vi "Command Injection.vi"() -> ()   [LabVIEW 2023]
doc: "Provides an example implementation of the Hardware Abstraction Framework to allow any attached instrument to be queried for its identity. The instrument must implement the SCPI standard.\n\nThe example application is clearly overly complex for the simple purpose of obtaining identity. However, it has been written to show how complex applications can be derived using the provided Event-Process-Result Handling mechanism. In fact, the base application can be reused by replacing the \"App ActionX Process\" VIs and \"Result Handling VIs\" as needed.\n\nNote that this example is just one way of interacting with the Framework. Ultimately, you just need to set up a Test Processor with what is needed and tell it to \"Process Directors\"."
uses:
  ReadCommand/ReadCommand.lvclass
  All Internal Message Ids.ctl
  ResourceEnumerator/ResourceEnumerator.lvclass
  InteractionProcessor/InteractionProcessor.lvclass
  CommandDirector/CommandDirector.lvclass
  <extravilib>/ChannelInstances/Tag-bool/Read With Abort.vi
  <extravilib>/ChannelInstances/Tag-bool/Write With Abort.vi
  <extravilib>/ChannelInstances/Tag-bool/Instantiate.vi
  <extravilib>/ChannelInstances/Tag-bool/EndpointRead.vi
  <extravilib>/ChannelInstances/Tag-bool/Endpoint.vi
  HAF.lvlib
  <extravilib>/ChannelInstances/Tag-bool.lvlib
panel:
  out "DC Read":u32
  out "DC Write":i32
  out "Read Duty Cycle":i32(slide) min=0 max=4095 step=1 scale=0.0..4095.0
  in  "Set Duty Cycle":i32(slide)=1007 max=4095 step=1 scale=0.0..4095.0
  in  "Pin":u8 max=7 step=1
  out "error out":errorcluster
  out "IDs":string[](array[string])
  out "Running":bool
  in  "Action10":bool
  in  "Action9":bool
  in  "Action8":bool
  in  "Action7":bool
  in  "Action6":bool
  in  "Action5":bool
  in  "Action4":bool
  in  "Action3":bool
  in  "Action2":bool
  in  "Instruments 2":string(combo)
  in  "Resume":bool
  in  "Pause":bool
  in  "Stop":bool
  in  "Start":bool caption="Action1"
  out "Instrument Id":string
  in  "Refresh":bool
  in  "Instruments":string(combo)
  # "Defined Behaviour Buttons"
  # "Command Injection - Pi Pico"
  # "Re-usable Controls\n\nThese are hidden at runtime.  Unhide if used."
  # "Provides an example implementation of the Hardware Abstraction Framework to show how Commands can be injected into an interaction whilst it is already running.  It uses a Raspberry Pi Pico with firmware developed by Jan Cumps and Shabaz available at \nhttps://github.com/jancumps/pico_scpi_usbtmc_labtool/releases/tag/v0.2.1\n\nOnce running, ensure the Pi Pico is selected in the Instruments drop down list then click Start.  Select a pin and move the gauge labelled \"Set Duty Cycle\" to inject commands to write the new value to the Pi and then read the pin. \n\nThe application starts the interaction running with one CommandDirector to get the ID from the Pico.  Normally this would then end the interaction (it's a run-once Director) but the InteractionProcessor is set to Handle Injections which prevents it terminating until Stop is pressed.  Each time the Set Duty Cycle gauge is moved it generates a UI event in the Event Loop which messages the Main Processing Loop to inject the commands.  \n\nThe VI is terminated by clicking on Stop."
  # "Defined Behaviour Buttons\n\nDrag the control from here to where needed.  You can relabel them but their behaviour is fixed in the application.\nYou may change this behaviour as well of course.\nStop and Refresh have been used."
  # "Instruments"
  # "Action Buttons"
  # "Instruments\n\nThese hold a list of Instruments attached to the PC and are populated by the \"Refresh\" Process case.  The Refresh button re-populates them."
  # "Action  Buttons\n\nDrag the control from here to where you need them on your panel.  Re-label and add button text as desired.\n\nPut processing code in the Process Case under their caption value.\n\nAction1 has been used and named \"Get Id\""
  # "="
  # "Other"
  # "Other\n\nOther potentially useful controls or indicators. \nIDs is the collection of UUIDs generated for Commands during execution.\nThe LED Running is used in this example."
  # "="
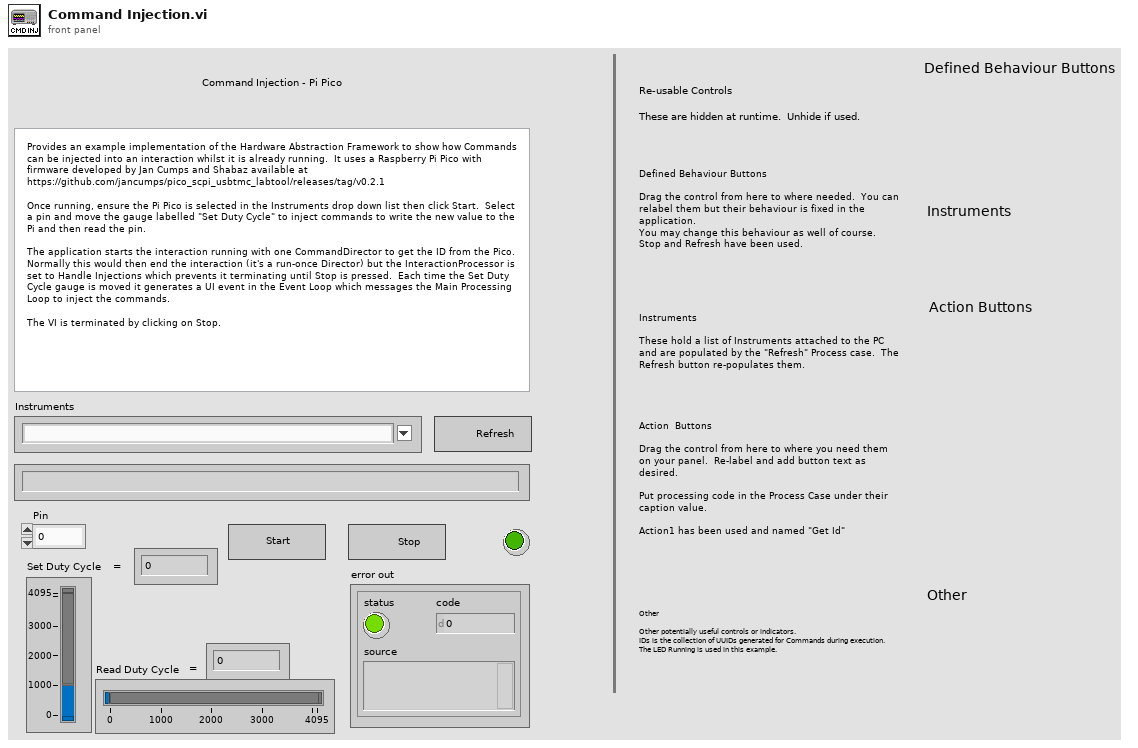
[diagram p1: front panel]
types:
  T1 = typedef "HAF.lvlib/All Message Queues.ctl" = cluster{"Internal":refnum<queue>, "Notifications":refnum<queue>}
  T2 = typedef "HAF.lvlib/All Events.ctl" = cluster{"Stop":T3, "Pause":T4, "Resume":T5, "Done":T6, "Injection":T7}
  T3 = typedef "HAF.lvlib/Stop Event.ctl" = refnum<user-event>
  T4 = typedef "HAF.lvlib/Pause Event.ctl" = refnum<user-event>
  T5 = typedef "HAF.lvlib/Resume Event.ctl" = refnum<user-event>
  T6 = typedef "HAF.lvlib/Done Event.ctl" = refnum<user-event>
  T7 = typedef "HAF.lvlib/Injection Event.ctl" = refnum<user-event>
  T8 = typedef "HAF.lvlib/All Internal Message Ids.ctl" = cluster{"Initialise":string, "Process":string, "Continue":string, "Done":string, "Pause":string, "Resume":string, "Stop":string, "Exit":string, "Inject":string}
  T9 = typedef "Tag-bool.lvlib/))Channel.ctl" = refnum<queue>
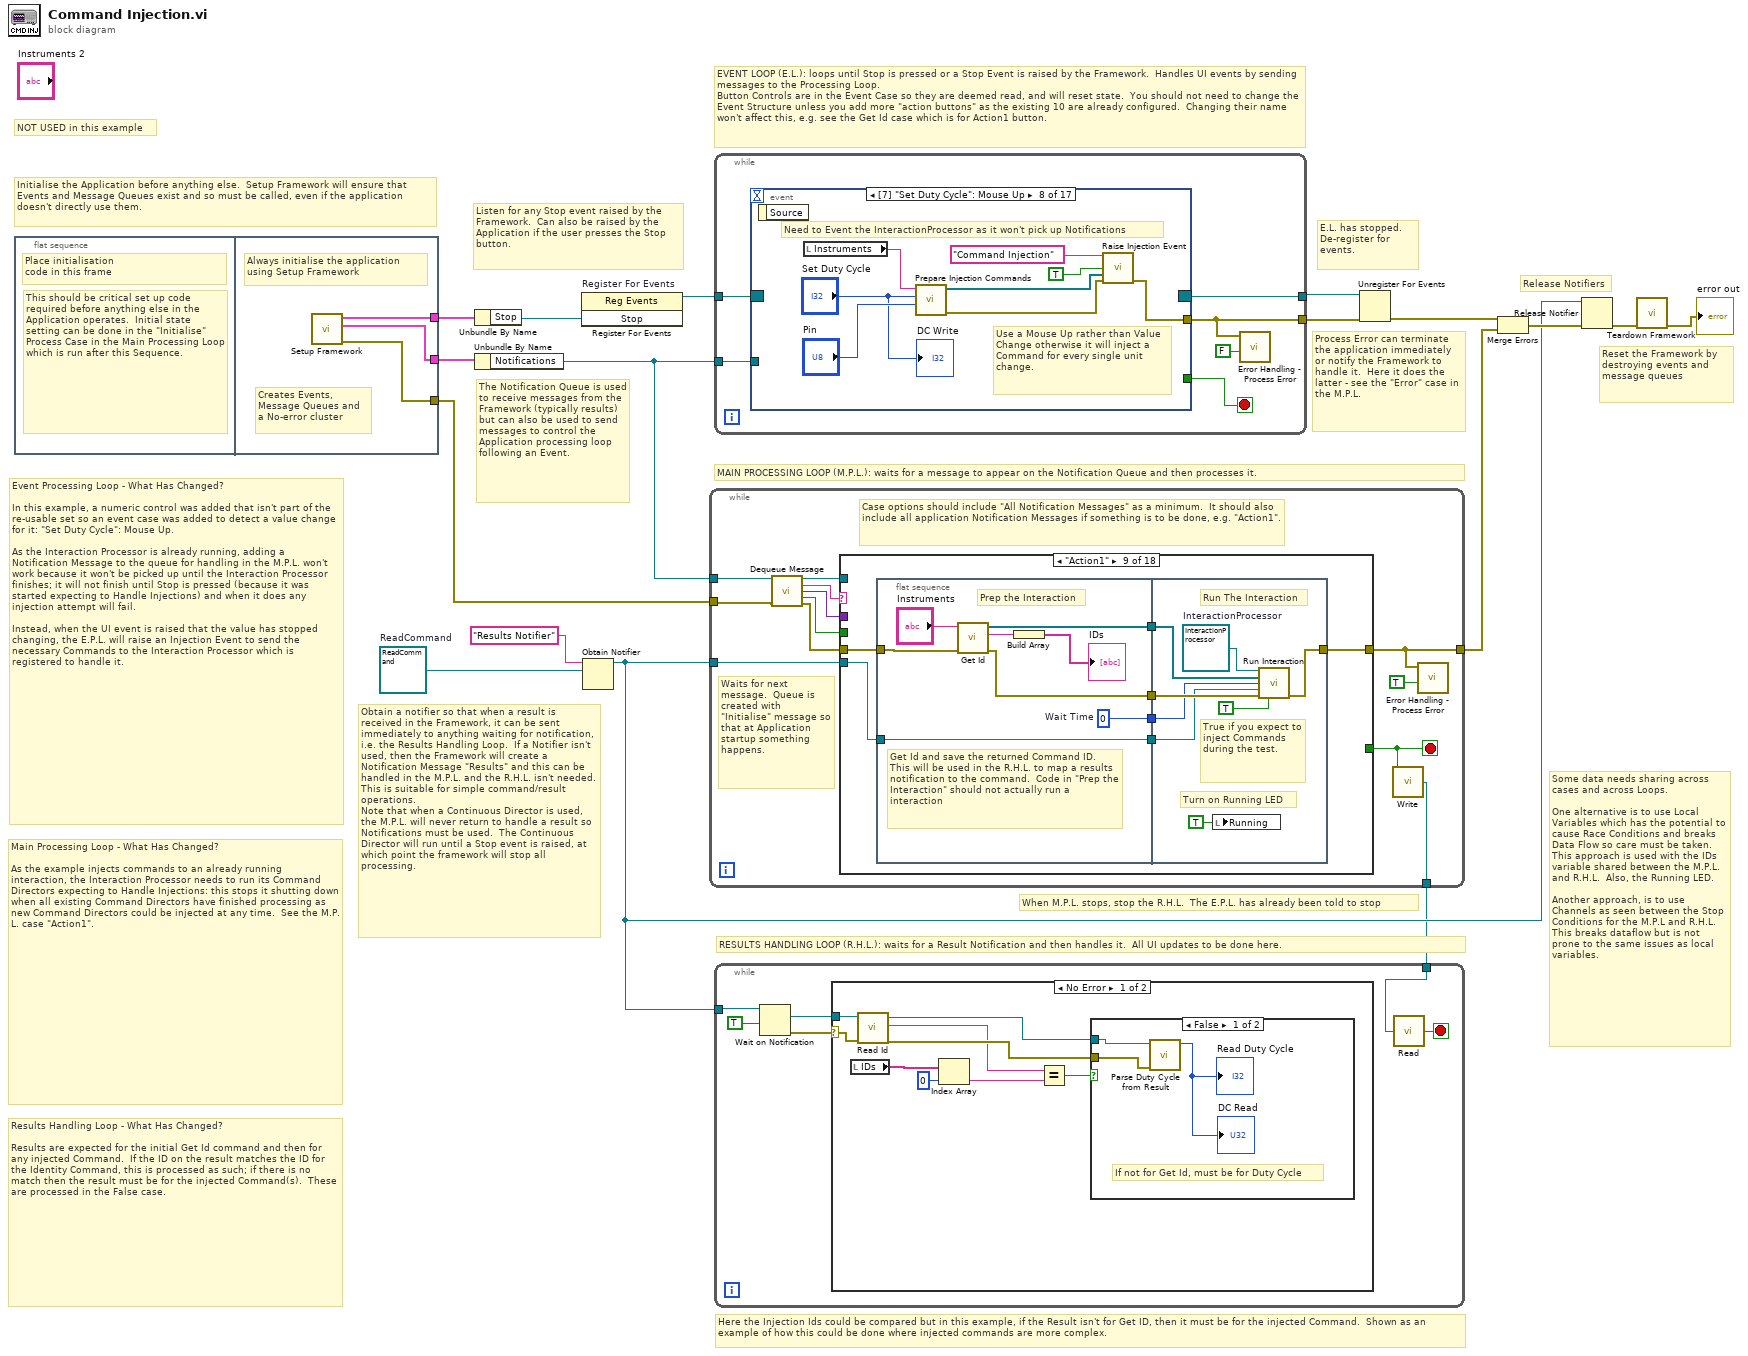
[diagram p0: block diagram]
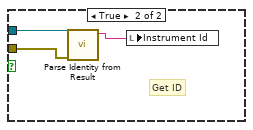
[diagram p2: hidden frame]
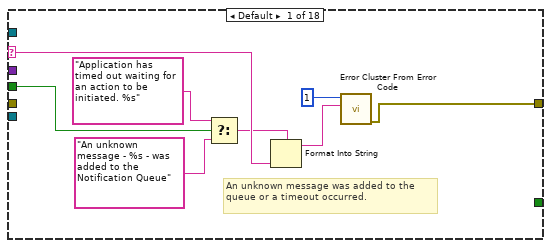
[diagram p4: hidden frame]
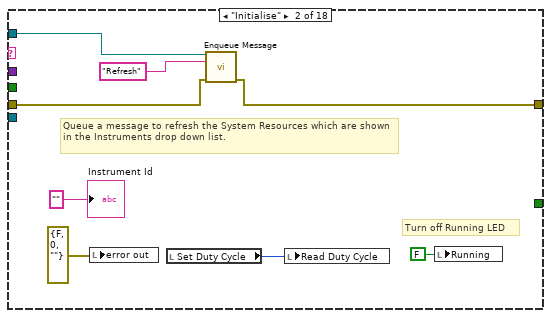
[diagram p5: hidden frame]
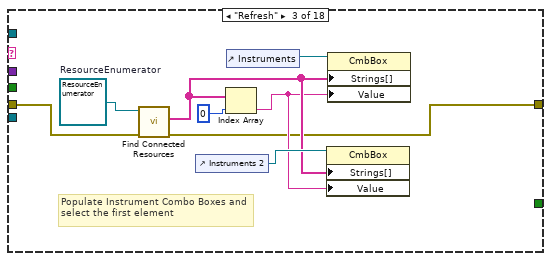
[diagram p6: hidden frame]
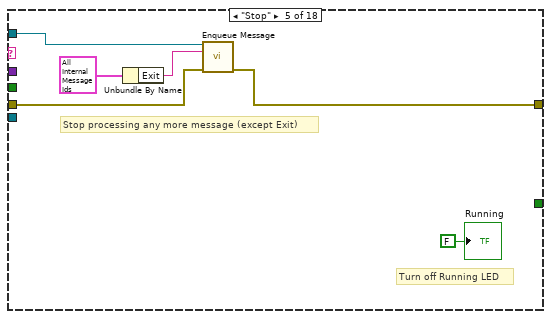
[diagram p8: hidden frame]
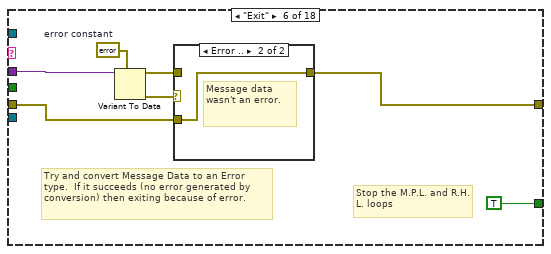
[diagram p9: hidden frame]
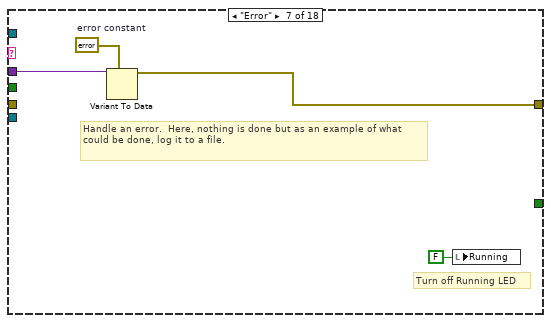
[diagram p11: hidden frame]
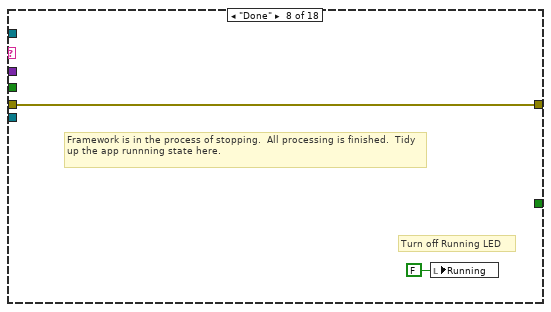
[diagram p12: hidden frame]
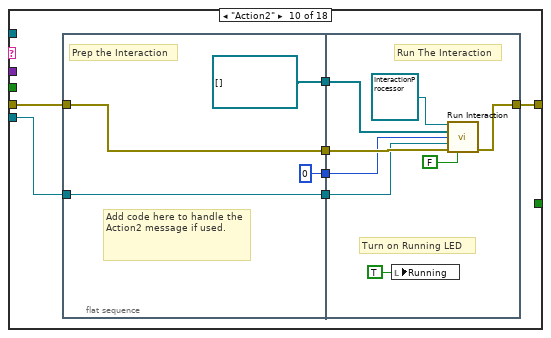
[diagram p13: hidden frame]
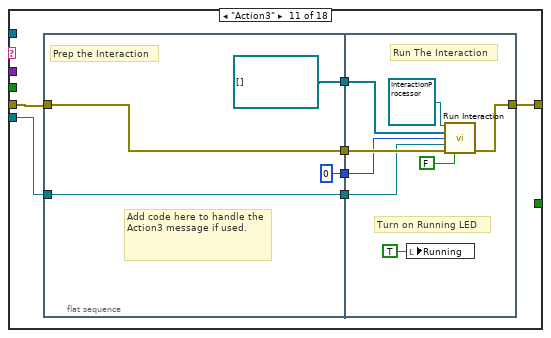
[diagram p14: hidden frame]
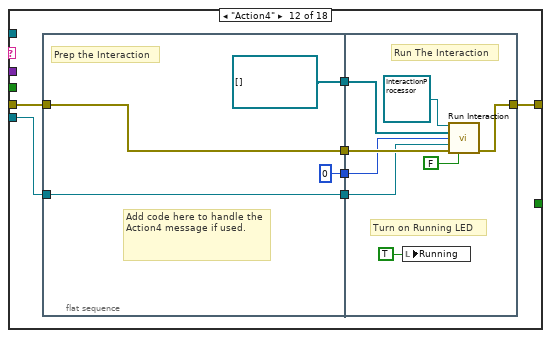
[diagram p15: hidden frame]
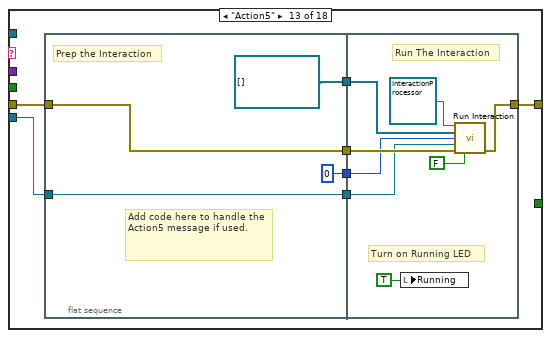
[diagram p16: hidden frame]
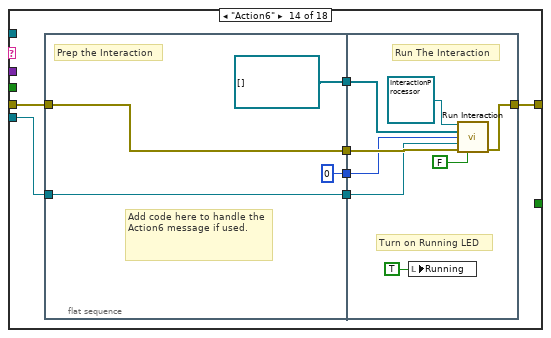
[diagram p17: hidden frame]
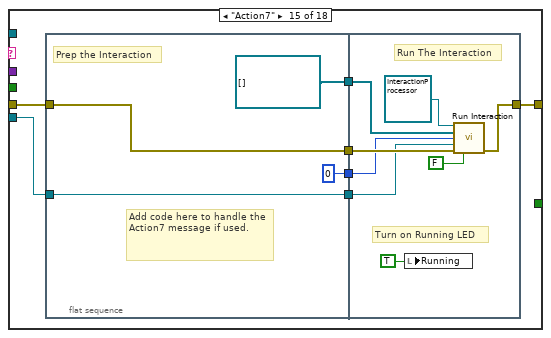
[diagram p18: hidden frame]
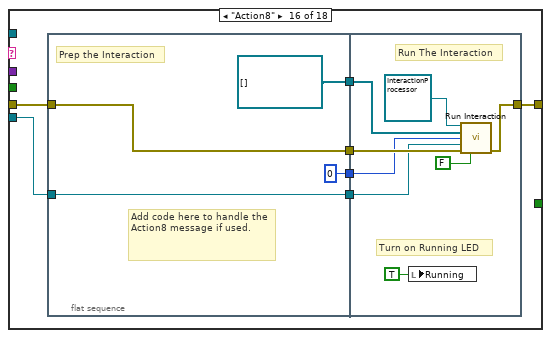
[diagram p19: hidden frame]
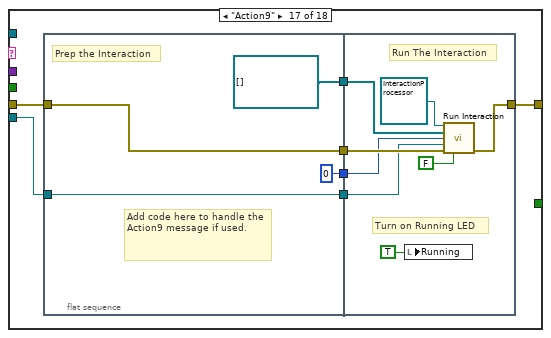
[diagram p20: hidden frame]
diagram:
  w8 = refnum<class "ReadCommand.lvclass"> refnum  # ReadCommand
  # "Here the Injection Ids could be compared but in this example, if the Result isn't for Get ID, then it must be for the injected Command.  Shown as an example of how this could be done where injected commands are more complex."
  # "When M.P.L. stops, stop the R.H.L.  The E.P.L. has already been told to stop"
  # "Results Handling Loop - What Has Changed?\n\nResults are expected for the initial Get Id command and then for any injected Command.  If the ID on the result matches the ID for the Identity Command, this is processed as such; if there is no match then the result must be for the injected Command(s).  These are processed in the False case."
  # "Reset the Framework by destroying events and message queues"
  # "Release Notifiers"
  # "Main Processing Loop - What Has Changed?\n\nAs the example injects commands to an already running interaction, the Interaction Processor needs to run its Command Directors expecting to Handle Injections: this stops it shutting down when all existing Command Directors have finished processing as new Command Directors could be injected at any time.  See the M.P.L. case \"Action1\"."
  # "Event Processing Loop - What Has Changed?\n\nIn this example, a numeric control was added that isn't part of the re-usable set so an event case was added to detect a value change for it: \"Set Duty Cycle\": Mouse Up.\n\nAs the Interaction Processor is already running, adding a Notification Message to the queue for handling in the M.P.L. won't work because it won't be picked up until the Interaction Processor finishes; it will not finish until Stop is pressed (because it was started expecting to Handle Injections) and when it does any injection attempt will fail.\n\nInstead, when the UI event is raised that the value has stopped changing, the E.P.L. will raise an Injection Event to send the necessary Commands to the Interaction Processor which is registered to handle it."
  # "Some data needs sharing across cases and across Loops.\n\nOne alternative is to use Local Variables which has the potential to cause Race Conditions and breaks Data Flow so care must be taken.  This approach is used with the IDs variable shared between the M.P.L. and R.H.L.  Also, the Running LED.\n\nAnother approach, is to use Channels as seen between the Stop Conditions for the M.P.L and R.H.L.  This breaks dataflow but is not prone to the same issues as local variables."
  # "Obtain a notifier so that when a result is received in the Framework, it can be sent immediately to anything waiting for notification, i.e. the Results Handling Loop.  If a Notifier isn't used, then the Framework will create a Notification Message \"Results\" and this can be handled in the M.P.L. and the R.H.L. isn't needed.  This is suitable for simple command/result operations.\nNote that when a Continuous Director is used, the M.P.L. will never return to handle a result so Notifications must be used.  The Continuous Director will run until a Stop event is raised, at which point the framework will stop all processing."
  # "Process Error can terminate the application immediately or notify the Framework to handle it.  Here it does the latter - see the \"Error\" case in the M.P.L."
  # "E.L. has stopped.  De-register for events."
  # "RESULTS HANDLING LOOP (R.H.L.): waits for a Result Notification and then handles it.  All UI updates to be done here."
  # "MAIN PROCESSING LOOP (M.P.L.): waits for a message to appear on the Notification Queue and then processes it."
  # "EVENT LOOP (E.L.): loops until Stop is pressed or a Stop Event is raised by the Framework.  Handles UI events by sending messages to the Processing Loop.\nButton Controls are in the Event Case so they are deemed read, and will reset state.  You should not need to change the Event Structure unless you add more \"action buttons\" as the existing 10 are already configured.  Changing their name won't affect this, e.g. see the Get Id case which is for Action1 button."
  # "NOT USED in this example"
  # "Listen for any Stop event raised by the Framework.  Can also be raised by the Application if the user presses the Stop button."
  # "The Notification Queue is used to receive messages from the Framework (typically results) but can also be used to send messages to control the Application processing loop following an Event."
  # "Initialise the Application before anything else.  Setup Framework will ensure that Events and Message Queues exist and so must be called, even if the application doesn't directly use them."
  n1 = flat-sequence {
    tunnel: [w20] -> w16
    tunnel: [w19] -> w17
    tunnel: [w18] -> w10
    frame #0 {
      # "This should be critical set up code required before anything else in the Application operates.  Initial state setting can be done in the \"Initialise\" Process Case in the Main Processing Loop which is run after this Sequence."
      # "Place initialisation\ncode in this frame"
    }
    frame #1 {
      # "Creates Events,  \nMessage Queues and\na No-error cluster"
      # "Always initialise the application using Setup Framework"
      n2 = call "Setup Framework.vi"() -> ("error out"=w18:errorcluster, "Message Queues"=w19:T1, "Events"=w20:T2)  [unwired: 9 in]
    }
  }
  n3 = Unbundle By Name(w16) -> ("Stop"=w14:T3)
  n4 = Unbundle By Name(w17) -> ("Notifications"=w11:refnum<queue>)
  n5 = register-events "Register For Events"(w14) -> (reference out=w15:refnum<event-registration>)  [unwired: 2 in, 1 out]
  n6 = Obtain Notifier(name (unnamed)="Results Notifier", notification data type=w8) -> (notifier out=w4:refnum<notifier>)  [unwired: 2 in, 2 out]
  n7 = while {
    tunnel: w11 -> [w32]
    tunnel: w10 -> [w31]
    tunnel: w4 -> [w25]
    tunnel: [w24] -> w6
    tunnel: [w21] -> w1
    stop <- w22 stop-if-true
    # "Case options should include \"All Notification Messages\" as a minimum.  It should also include all application Notification Messages if something is to be done, e.g. \"Action1\"."
    # "Waits for next message.  Queue is created with \"Initialise\" message so that at Application startup something happens."
    n8 = call "Dequeue Message.vi"("Message Queue In"=w32, "error in (no error)"=w31) -> ("Message Queue Out"=w30:refnum<queue>, "Message Id"=w29:string, "Message Data"=w28:variant, "Timed Out"=w26:bool, "error out"=w27:errorcluster)  [unwired: 9 in]
    n9 = case shown="\"Action1\"" w29 {
      selector: w29 -> [w37 _ _ _ _ _ _ _ _ _ _ _ _ _ _ _ _ _]
      tunnel: w30 -> [_ w48 _ _ w63 _ _ _ _ _ _ _ _ _ _ _ _ _]
      tunnel: w28 -> [_ _ _ _ _ w70 w76 _ _ _ _ _ _ _ _ _ _ _]
      tunnel: w27 -> [_ w46 w55 w57 w60 w66 _ w78 w84 w104 w122 w140 w160 w179 w198 w217 w237 w255]
      tunnel: w26 -> [w39 _ _ _ _ _ _ _ _ _ _ _ _ _ _ _ _ _]
      tunnel: w25 -> [_ _ _ _ _ _ _ _ w85 w103 w121 w141 w159 w178 w197 w216 w236 w254]
      tunnel: [w33 w45 w49 w57 w59 w67 w75 w78 w83 w102 w123 w142 w161 w180 w199 w218 w235 w256] -> w24
      tunnel: [_ _ _ _ _ TRUE ("Running") _ _ _ _ _ _ _ _ _ _ _ _] -> w22
      frame Default {
        # "An unknown message was added to the queue or a timeout occurred."
        n10 = Select(t="Application has timed out waiting for an action to be initiated. %s", s=w39, f="An unknown message - %s - was added to the Notification Queue") -> (s? t:f=w36:string)
        n11 = Format Into String(format string=w36, w37) -> (resulting string=w34:string)  [unwired: 2 in, 1 out]
        n12 = call <vilib>:"Error Cluster From Error Code.vi"("error message (\"\")"=w34, "error code (0)"=1) -> ("error out"=w33:errorcluster)  [unwired: 7 in]
      }
      frame "Initialise" {
        # "Turn off Running LED"
        # "Queue a message to refresh the System Resources which are shown in the Instruments drop down list."
        n13 = local write "error out"(errorcluster {"status"=FALSE, "code"=0, "source"=""} ("error constant")) -> ()
        n14 = local read "Set Duty Cycle"() -> (w41:i32)
        n15 = call "Enqueue Message.vi"("Message Queue In"=w48, "Message Id"="Refresh", "error in (no error)"=w46) -> ("error out"=w45:errorcluster)  [unwired: 11 in, 1 out]
        n16 = local write "Read Duty Cycle"(w41) -> ()
        n17 = local write "Running"(FALSE ("Running")) -> ()
        "Instrument Id" <- "" ("Instrument Id")
      }
      frame "Refresh" {
        w56 = refnum<class "ResourceEnumerator.lvclass"> refnum  # ResourceEnumerator
        # "Populate Instrument Combo Boxes and select the first element"
        n18 = call-dynamic "Find Connected Resources.vi"("error in (no error)"=w55, "AbstractResourceEnumerator in"=w56) -> ("error out"=w49:errorcluster, "Found Resources"=w51:string[])  [unwired: 7 in, 1 out]
        n19 = control-ref of="Instruments 2"() -> (w52:refnum<vi>)
        n20 = Index Array(array=w51, index=0) -> (element=w50:string)
        n21 = control-ref of="Instruments"() -> (w54:refnum<vi>)
        n22 = property class="CmbBox"(reference=w52, "Strings[]"=w51, "Value"=w50) -> ()  [unwired: 1 in, 2 out]
        n23 = property class="CmbBox"(reference=w54, "Strings[]"=w51, "Value"=w50) -> ()  [unwired: 1 in, 2 out]
      }
      frame "Results" {
        # "If a notifier isn't being used, then the framework will put the results onto the Notification Queue and should be handled here.  Note that this will only be available when the Interaction Processor has finished processing everything."
      }
      frame "Stop" {
        # "Stop processing any more message (except Exit)"
        # "Turn off Running LED"
        n24 = Unbundle By Name(T8 {"Initialise"="Initialise", "Process"="Process", "Continue"="Continue", "Done"="Done", "Pause"="Pause", "Resume"="Resume", "Stop"="Stop", "Exit"="Exit", "Inject"=""} ("Message Ids")) -> ("Exit"=w61:string)
        n25 = call "Enqueue Message.vi"("Message Queue In"=w63, "Message Id"=w61, "error in (no error)"=w60) -> ("error out"=w59:errorcluster)  [unwired: 11 in, 1 out]
        "Running" <- FALSE ("Running")
      }
      frame "Exit" {
        w65 = errorcluster {"status"=FALSE, "code"=0, "source"=""}  # error constant
        # "Try and convert Message Data to an Error type.  If it succeeds (no error generated by conversion) then exiting because of error."
        # "Stop the M.P.L. and R.H.L. loops"
        n26 = Variant To Data(type=w65, Variant=w70) -> (data=w68:errorcluster, error out=w69:errorcluster)  [unwired: 1 in]
        n27 = case shown="Error .." w69 {
          tunnel: w68 -> [w71 _]
          tunnel: [w71 w72] -> w67
          tunnel: w66 -> [_ w72]
          frame No Error {
            # "If exiting because of error, pass it on for display"
          }
          frame Error {
            # "Message data wasn't an error."
          }
        }
      }
      frame "Error" {
        w74 = errorcluster {"status"=FALSE, "code"=0, "source"=""}  # error constant
        # "Turn off Running LED"
        # "Handle an error.  Here, nothing is done but as an example of what could be done, log it to a file."
        n28 = Variant To Data(type=w74, Variant=w76) -> (data=w75:errorcluster)  [unwired: 1 in, 1 out]
        n29 = local write "Running"(FALSE ("Running")) -> ()
      }
      frame "Done" {
        # "Turn off Running LED"
        # "Framework is in the process of stopping.  All processing is finished.  Tidy up the app runnning state here."
        n30 = local write "Running"(FALSE ("Running")) -> ()
      }
      frame "Action1" {
        n31 = flat-sequence {
          tunnel: w85 -> [w87]
          tunnel: w84 -> [w92]
          tunnel: [w91] -> w82
          tunnel: [w88] -> w81
          tunnel: [w87] -> w80
          tunnel: [w86] -> w79
          tunnel: [w101] -> w83
          tunnel: w82 -> [w99]
          tunnel: w81 -> [w100]
          tunnel: w80 -> [w98]
          tunnel: w79 -> [w97]
          frame #0 {
            w86 = u32 0  # Wait Time
            # "Get Id and save the returned Command ID.  This will be used in the R.H.L. to map a results notification to the command.  Code in \"Prep the Interaction\" should not actually run a interaction"
            # "Prep the Interaction"
            n32 = call "Get Id.vi"("error in (no error)"=w92, "Instrument Name"="Instruments") -> ("error out"=w91:errorcluster, "ID of IDN Command"=w89:string, "CommandDirectors"=w88:refnum<class "CommandDirector.lvclass">[])  [unwired: 6 in]
            n33 = Build Array(w89) -> (→"IDs":string[])
          }
          frame #1 {
            w94 = refnum<class "InteractionProcessor.lvclass"> refnum  # InteractionProcessor
            # "True if you expect to inject Commands during the test."
            # "Turn on Running LED"
            # "Run The Interaction"
            n34 = local write "Running"(TRUE ("Running")) -> ()
            n35 = call-dynamic "Run Interaction.vi"("InteractionProcessor in"=w94, "Command Directors"=w100, "Wait Time"=w97, "Results Notifier"=w98, "error in (no error)"=w99, "Handle Injections"=TRUE) -> ("error out"=w101:errorcluster)  [unwired: 8 in, 1 out]
          }
        }
      }
      frame "Action2" {
        n36 = flat-sequence {
          tunnel: w103 -> [w112]
          tunnel: w104 -> [w111]
          tunnel: [w111] -> w108
          tunnel: [refnum<class "CommandDirector.lvclass">[] [] ("CommandDirectors")] -> w107
          tunnel: [w112] -> w106
          tunnel: [u32 0 ("Wait Time")] -> w105
          tunnel: [w120] -> w102
          tunnel: w108 -> [w118]
          tunnel: w107 -> [w119]
          tunnel: w106 -> [w117]
          tunnel: w105 -> [w116]
          frame #0 {
            # "Add code here to handle the Action2 message if used."
            # "Prep the Interaction"
          }
          frame #1 {
            # "Turn on Running LED"
            # "Run The Interaction"
            n37 = local write "Running"(TRUE ("Running")) -> ()
            n38 = call-dynamic "Run Interaction.vi"("InteractionProcessor in"=refnum<class "InteractionProcessor.lvclass"> refnum ("InteractionProcessor"), "Command Directors"=w119, "Wait Time"=w116, "Results Notifier"=w117, "error in (no error)"=w118, "Handle Injections"=FALSE) -> ("error out"=w120:errorcluster)  [unwired: 8 in, 1 out]
          }
        }
      }
      frame "Action3" {
        n39 = flat-sequence {
          tunnel: w121 -> [w131]
          tunnel: w122 -> [w130]
          tunnel: [w130] -> w127
          tunnel: [refnum<class "CommandDirector.lvclass">[] [] ("CommandDirectors")] -> w126
          tunnel: [w131] -> w125
          tunnel: [u32 0 ("Wait Time")] -> w124
          tunnel: [w139] -> w123
          tunnel: w127 -> [w137]
          tunnel: w126 -> [w138]
          tunnel: w125 -> [w136]
          tunnel: w124 -> [w135]
          frame #0 {
            # "Add code here to handle the Action3 message if used."
            # "Prep the Interaction"
          }
          frame #1 {
            # "Turn on Running LED"
            # "Run The Interaction"
            n40 = local write "Running"(TRUE ("Running")) -> ()
            n41 = call-dynamic "Run Interaction.vi"("InteractionProcessor in"=refnum<class "InteractionProcessor.lvclass"> refnum ("InteractionProcessor"), "Command Directors"=w138, "Wait Time"=w135, "Results Notifier"=w136, "error in (no error)"=w137, "Handle Injections"=FALSE) -> ("error out"=w139:errorcluster)  [unwired: 8 in, 1 out]
          }
        }
      }
      frame "Action4" {
        n42 = flat-sequence {
          tunnel: w141 -> [w150]
          tunnel: w140 -> [w149]
          tunnel: [w149] -> w146
          tunnel: [refnum<class "CommandDirector.lvclass">[] [] ("CommandDirectors")] -> w145
          tunnel: [w150] -> w144
          tunnel: [u32 0 ("Wait Time")] -> w143
          tunnel: [w158] -> w142
          tunnel: w146 -> [w156]
          tunnel: w145 -> [w157]
          tunnel: w144 -> [w155]
          tunnel: w143 -> [w154]
          frame #0 {
            # "Add code here to handle the Action4 message if used."
            # "Prep the Interaction"
          }
          frame #1 {
            # "Turn on Running LED"
            # "Run The Interaction"
            n43 = local write "Running"(TRUE ("Running")) -> ()
            n44 = call-dynamic "Run Interaction.vi"("InteractionProcessor in"=refnum<class "InteractionProcessor.lvclass"> refnum ("InteractionProcessor"), "Command Directors"=w157, "Wait Time"=w154, "Results Notifier"=w155, "error in (no error)"=w156, "Handle Injections"=FALSE) -> ("error out"=w158:errorcluster)  [unwired: 8 in, 1 out]
          }
        }
      }
      frame "Action5" {
        n45 = flat-sequence {
          tunnel: w159 -> [w169]
          tunnel: w160 -> [w168]
          tunnel: [w168] -> w165
          tunnel: [refnum<class "CommandDirector.lvclass">[] [] ("CommandDirectors")] -> w164
          tunnel: [w169] -> w163
          tunnel: [u32 0 ("Wait Time")] -> w162
          tunnel: [w177] -> w161
          tunnel: w165 -> [w175]
          tunnel: w164 -> [w176]
          tunnel: w163 -> [w174]
          tunnel: w162 -> [w173]
          frame #0 {
            # "Add code here to handle the Action5 message if used."
            # "Prep the Interaction"
          }
          frame #1 {
            # "Turn on Running LED"
            # "Run The Interaction"
            n46 = local write "Running"(TRUE ("Running")) -> ()
            n47 = call-dynamic "Run Interaction.vi"("InteractionProcessor in"=refnum<class "InteractionProcessor.lvclass"> refnum ("InteractionProcessor"), "Command Directors"=w176, "Wait Time"=w173, "Results Notifier"=w174, "error in (no error)"=w175, "Handle Injections"=FALSE) -> ("error out"=w177:errorcluster)  [unwired: 8 in, 1 out]
          }
        }
      }
      frame "Action6" {
        n48 = flat-sequence {
          tunnel: w178 -> [w188]
          tunnel: w179 -> [w187]
          tunnel: [w187] -> w184
          tunnel: [refnum<class "CommandDirector.lvclass">[] [] ("CommandDirectors")] -> w183
          tunnel: [w188] -> w182
          tunnel: [u32 0 ("Wait Time")] -> w181
          tunnel: [w196] -> w180
          tunnel: w184 -> [w194]
          tunnel: w183 -> [w195]
          tunnel: w182 -> [w193]
          tunnel: w181 -> [w192]
          frame #0 {
            # "Add code here to handle the Action6 message if used."
            # "Prep the Interaction"
          }
          frame #1 {
            # "Turn on Running LED"
            # "Run The Interaction"
            n49 = local write "Running"(TRUE ("Running")) -> ()
            n50 = call-dynamic "Run Interaction.vi"("InteractionProcessor in"=refnum<class "InteractionProcessor.lvclass"> refnum ("InteractionProcessor"), "Command Directors"=w195, "Wait Time"=w192, "Results Notifier"=w193, "error in (no error)"=w194, "Handle Injections"=FALSE) -> ("error out"=w196:errorcluster)  [unwired: 8 in, 1 out]
          }
        }
      }
      frame "Action7" {
        n51 = flat-sequence {
          tunnel: w197 -> [w207]
          tunnel: w198 -> [w206]
          tunnel: [w206] -> w203
          tunnel: [refnum<class "CommandDirector.lvclass">[] [] ("CommandDirectors")] -> w202
          tunnel: [w207] -> w201
          tunnel: [u32 0 ("Wait Time")] -> w200
          tunnel: [w215] -> w199
          tunnel: w203 -> [w213]
          tunnel: w202 -> [w214]
          tunnel: w201 -> [w212]
          tunnel: w200 -> [w211]
          frame #0 {
            # "Add code here to handle the Action7 message if used."
            # "Prep the Interaction"
          }
          frame #1 {
            # "Turn on Running LED"
            # "Run The Interaction"
            n52 = local write "Running"(TRUE ("Running")) -> ()
            n53 = call-dynamic "Run Interaction.vi"("InteractionProcessor in"=refnum<class "InteractionProcessor.lvclass"> refnum ("InteractionProcessor"), "Command Directors"=w214, "Wait Time"=w211, "Results Notifier"=w212, "error in (no error)"=w213, "Handle Injections"=FALSE) -> ("error out"=w215:errorcluster)  [unwired: 8 in, 1 out]
          }
        }
      }
      frame "Action8" {
        n54 = flat-sequence {
          tunnel: w216 -> [w226]
          tunnel: w217 -> [w225]
          tunnel: [w225] -> w222
          tunnel: [refnum<class "CommandDirector.lvclass">[] [] ("CommandDirectors")] -> w221
          tunnel: [w226] -> w220
          tunnel: [u32 0 ("Wait Time")] -> w219
          tunnel: [w234] -> w218
          tunnel: w222 -> [w232]
          tunnel: w221 -> [w233]
          tunnel: w220 -> [w231]
          tunnel: w219 -> [w230]
          frame #0 {
            # "Add code here to handle the Action8 message if used."
            # "Prep the Interaction"
          }
          frame #1 {
            # "Turn on Running LED"
            # "Run The Interaction"
            n55 = local write "Running"(TRUE ("Running")) -> ()
            n56 = call-dynamic "Run Interaction.vi"("InteractionProcessor in"=refnum<class "InteractionProcessor.lvclass"> refnum ("InteractionProcessor"), "Command Directors"=w233, "Wait Time"=w230, "Results Notifier"=w231, "error in (no error)"=w232, "Handle Injections"=FALSE) -> ("error out"=w234:errorcluster)  [unwired: 8 in, 1 out]
          }
        }
      }
      frame "Action9" {
        n57 = flat-sequence {
          tunnel: w236 -> [w245]
          tunnel: w237 -> [w244]
          tunnel: [w244] -> w241
          tunnel: [refnum<class "CommandDirector.lvclass">[] [] ("CommandDirectors")] -> w240
          tunnel: [w245] -> w239
          tunnel: [u32 0 ("Wait Time")] -> w238
          tunnel: w241 -> [w252]
          tunnel: w240 -> [w253]
          tunnel: w239 -> [w251]
          tunnel: w238 -> [w250]
          tunnel: [w249] -> w235
          frame #0 {
            # "Add code here to handle the Action9 message if used."
            # "Prep the Interaction"
          }
          frame #1 {
            # "Turn on Running LED"
            # "Run The Interaction"
            n58 = local write "Running"(TRUE ("Running")) -> ()
            n59 = call-dynamic "Run Interaction.vi"("InteractionProcessor in"=refnum<class "InteractionProcessor.lvclass"> refnum ("InteractionProcessor"), "Command Directors"=w253, "Wait Time"=w250, "Results Notifier"=w251, "error in (no error)"=w252, "Handle Injections"=FALSE) -> ("error out"=w249:errorcluster)  [unwired: 8 in, 1 out]
          }
        }
      }
      frame "Action10" {
        n60 = flat-sequence {
          tunnel: w254 -> [w264]
          tunnel: w255 -> [w263]
          tunnel: [w263] -> w260
          tunnel: [refnum<class "CommandDirector.lvclass">[] [] ("CommandDirectors")] -> w259
          tunnel: [w264] -> w258
          tunnel: [u32 0 ("Wait Time")] -> w257
          tunnel: [w272] -> w256
          tunnel: w260 -> [w270]
          tunnel: w259 -> [w271]
          tunnel: w258 -> [w269]
          tunnel: w257 -> [w268]
          frame #0 {
            # "Add code here to handle the Action10 message if used."
            # "Prep the Interaction"
          }
          frame #1 {
            # "Turn on Running LED"
            # "Run The Interaction"
            n61 = local write "Running"(TRUE ("Running")) -> ()
            n62 = call-dynamic "Run Interaction.vi"("InteractionProcessor in"=refnum<class "InteractionProcessor.lvclass"> refnum ("InteractionProcessor"), "Command Directors"=w271, "Wait Time"=w268, "Results Notifier"=w269, "error in (no error)"=w270, "Handle Injections"=FALSE) -> ("error out"=w272:errorcluster)  [unwired: 8 in, 1 out]
          }
        }
      }
    }
    n63 = call <extravilib>:"Write.vi"("element"=w22) -> ("channel"=w21:T9)  [unwired: 1 out]
    n64 = call "Error Handling - Process Error.vi"("Exit on Error"=TRUE, "error to process"=w24) -> ()  [unwired: 9 in, 1 out]
  }
  n65 = while {
    tunnel: w11 -> [w277]
    tunnel: w15 -> [w278]
    tunnel: [w275] -> w13
    tunnel: [w274] -> w12
    stop <- w276 stop-if-true
    n66 = event shown="[7] \"Set Duty Cycle\": Mouse Up" {
      selector: w278 -> [_ _ _ _ _ _ _ _ _ _ _ _ _ _ _ _ _]
      dyn-events: [_ _ _ _ _ _ _ _ _ _ _ _ _ _ _ _ _] -> w275
      timeout: _ -> [_ _ _ _ _ _ _ _ _ _ _ _ _ _ _ _ _]
      tunnel: w277 -> [_ w281 _ _ w291 _ w299 _ w309 w312 w315 w318 w321 w324 w327 w330 w333]
      tunnel: [_ w279 w282 w285 w289 w294 w297 w307 w308 w311 w314 w317 w320 w323 w326 w329 w332] -> w274
      tunnel: [_ _ _ _ TRUE _ _ _ _ _ _ _ _ _ _ _ _] -> w276
      event Timeout {
        n67 = event-data() -> ()  [unwired: 1 in, 3 out]
      }
      event "Refresh": Value Change {
        # "Notify M.P.L. to rebuild attached instruments"
        n68 = event-data() -> ()  [unwired: 1 in, 1 out]
        n69 = call "Enqueue Message.vi"("Message Queue In"=w281, "Message Id"="Refresh") -> ("error out"=w279:errorcluster)  [unwired: 12 in, 1 out]
      }
      event "Pause": Value Change {
        # "Tell the Framework to Pause processing."
        n70 = event-data() -> ()  [unwired: 1 in, 1 out]
        n71 = call "Raise Pause Event.vi"("Raiser Name"="Command Injection", "Send Pause"=TRUE) -> ("error out"=w282:errorcluster)  [unwired: 8 in]
      }
      event "Resume": Value Change {
        # "Tell the Framework to Resume processing."
        n72 = event-data() -> ()  [unwired: 1 in, 1 out]
        n73 = call "Raise Resume Event.vi"("Send Resume"=TRUE, "Raiser Name"="Command Injection") -> ("error out"=w285:errorcluster)  [unwired: 9 in]
      }
      event User Event {
        # "Tell M.P.L. to stop processsing, high priority.  Exit Event Loop."
        n74 = event-data() -> ()  [unwired: 1 in, 1 out]
        n75 = Unbundle By Name(T8 {"Initialise"="Initialise", "Process"="Process", "Continue"="Continue", "Done"="Done", "Pause"="Pause", "Resume"="Resume", "Stop"="Stop", "Exit"="Exit", "Inject"=""} ("Message Ids")) -> ("Stop"=w292:string)
        n76 = call "Enqueue Message.vi"("Message Queue In"=w291, "Message Id"=w292, "Priority"=TRUE) -> ("error out"=w289:errorcluster)  [unwired: 11 in, 1 out]
      }
      event "Stop": Value Change {
        # "When Stop pressed, raise Stop Event to halt further processing"
        n77 = event-data() -> ()  [unwired: 1 in, 1 out]
        n78 = call "Raise Stop Event.vi"("Send Stop"=TRUE, "Raiser Name"="Command Injection") -> ("error out"=w294:errorcluster)  [unwired: 9 in]
      }
      event "Start": Value Change {
        # "ACTION 1 BTN"
        n79 = event-data() -> ()  [unwired: 1 in, 1 out]
        n80 = call "Enqueue Message.vi"("Message Queue In"=w299, "Message Id"="Action1") -> ("error out"=w297:errorcluster)  [unwired: 12 in, 1 out]
      }
      event "Set Duty Cycle": Mouse Up {
        # "Need to Event the InteractionProcessor as it won't pick up Notifications"
        # "Use a Mouse Up rather than Value Change otherwise it will inject a Command for every single unit change."
        n81 = event-data() -> ()  [unwired: 1 in, 1 out]
        n82 = local read "Instruments"() -> (w306:string)
        n83 = call "Prepare Injection Commands.vi"("Pin"="Pin", "Duty Cycle"="Set Duty Cycle", "Instrument Name"=w306) -> ("error out"=w303:errorcluster, "Injection Commands"=w302:refnum<class "CommandDirector.lvclass">[])  [unwired: 6 in, 1 out]
        n84 = call "Raise Injection Event.vi"("Raiser Name"="Command Injection", "Send Injection"=TRUE, "Injected Command Directors"=w302, "error in (no error)"=w303) -> ("error out"=w307:errorcluster)  [unwired: 11 in]
        "DC Write" <- "Set Duty Cycle"
      }
      event "Action2": Value Change {
        # "ACTION 2 BTN"
        n85 = event-data() -> ()  [unwired: 1 in, 1 out]
        n86 = call "Enqueue Message.vi"("Message Queue In"=w309, "Message Id"="Action2") -> ("error out"=w308:errorcluster)  [unwired: 12 in, 1 out]
      }
      event "Action3": Value Change {
        # "ACTION 3 BTN"
        n87 = event-data() -> ()  [unwired: 1 in, 1 out]
        n88 = call "Enqueue Message.vi"("Message Queue In"=w312, "Message Id"="Action3") -> ("error out"=w311:errorcluster)  [unwired: 12 in, 1 out]
      }
      event "Action4": Value Change {
        # "ACTION 4 BTN"
        n89 = event-data() -> ()  [unwired: 1 in, 1 out]
        n90 = call "Enqueue Message.vi"("Message Queue In"=w315, "Message Id"="Action4") -> ("error out"=w314:errorcluster)  [unwired: 12 in, 1 out]
      }
      event "Action5": Value Change {
        # "ACTION 5 BTN"
        n91 = event-data() -> ()  [unwired: 1 in, 1 out]
        n92 = call "Enqueue Message.vi"("Message Queue In"=w318, "Message Id"="Action5") -> ("error out"=w317:errorcluster)  [unwired: 12 in, 1 out]
      }
      event "Action6": Value Change {
        # "ACTION 6 BTN"
        n93 = event-data() -> ()  [unwired: 1 in, 1 out]
        n94 = call "Enqueue Message.vi"("Message Queue In"=w321, "Message Id"="Action6") -> ("error out"=w320:errorcluster)  [unwired: 12 in, 1 out]
      }
      event "Action7": Value Change {
        # "ACTION 7 BTN"
        n95 = event-data() -> ()  [unwired: 1 in, 1 out]
        n96 = call "Enqueue Message.vi"("Message Queue In"=w324, "Message Id"="Action7") -> ("error out"=w323:errorcluster)  [unwired: 12 in, 1 out]
      }
      event "Action8": Value Change {
        # "ACTION 8 BTN"
        n97 = event-data() -> ()  [unwired: 1 in, 1 out]
        n98 = call "Enqueue Message.vi"("Message Queue In"=w327, "Message Id"="Action8") -> ("error out"=w326:errorcluster)  [unwired: 12 in, 1 out]
      }
      event "Action9": Value Change {
        # "ACTION 9 BTN"
        n99 = event-data() -> ()  [unwired: 1 in, 1 out]
        n100 = call "Enqueue Message.vi"("Message Queue In"=w330, "Message Id"="Action9") -> ("error out"=w329:errorcluster)  [unwired: 12 in, 1 out]
      }
      event "Action10": Value Change {
        # "ACTION 10 BTN"
        n101 = event-data() -> ()  [unwired: 1 in, 1 out]
        n102 = call "Enqueue Message.vi"("Message Queue In"=w333, "Message Id"="Action1") -> ("error out"=w332:errorcluster)  [unwired: 12 in, 1 out]
      }
    }
    n103 = call "Error Handling - Process Error.vi"("Exit on Error"=FALSE, "error to process"=w274) -> ()  [unwired: 9 in, 1 out]
  }
  n104 = while {
    tunnel: w4 -> [w340]
    tunnel: w1 -> [w336]
    stop <- w337 stop-if-true
    n105 = Wait on Notification(notifier=w340, ignore previous (F)=TRUE) -> (notification=w339:refnum<class "ReadCommand.lvclass">, error out=w338:errorcluster)  [unwired: 2 in, 2 out]
    n106 = case shown="No Error" w338 {
      selector: w338 -> [w345 _]
      tunnel: w339 -> [w349 _]
      frame No Error {
        n107 = local read "IDs"() -> (w344:string[])
        n108 = call-dynamic "Read Id.vi"("error in (no error)"=w345, "WriteCommand in"=w349) -> ("error out"=w343:errorcluster, "Id"=w341:string, "WriteCommand out"=w342:refnum<class "ReadCommand.lvclass">)  [unwired: 7 in]
        n109 = Index Array(array=w344, index=0) -> (element=w347:string)
        n110 = Equal?(x=w341, y=w347) -> (x = y?=w346:bool)
        n111 = case shown="False" w346 {
          tunnel: w342 -> [w352 w355]
          tunnel: w343 -> [w351 w354]
          frame False {
            # "If not for Get Id, must be for Duty Cycle"
            n112 = call "Parse Duty Cycle from Result.vi"("error in (no error)"=w351, "ReadCommand In"=w352) -> ("Duty Cycle"=→"Read Duty Cycle" →"DC Read":i32)  [unwired: 8 in, 1 out]
          }
          frame True {
            # "Get ID"
            n113 = call "Parse Identity from Result.vi"("error in (no error)"=w354, "ReadCommand In"=w355) -> ("Identity"=w353:string)  [unwired: 8 in, 1 out]
            n114 = local write "Instrument Id"(w353) -> ()
          }
        }
      }
      frame Error {
      }
    }
    n115 = call <extravilib>:"Read.vi"("channel"=w336) -> ("element"=w337:bool)  [unwired: 1 in, 1 out]
  }
  n116 = Unregister For Events(event registration refnum=w13, error in=w12) -> (error out=w7:errorcluster)
  n117 = Merge Errors(w7, w6) -> (w5:errorcluster)
  n118 = Release Notifier(notifier=w4, error in (no error)=w5) -> (error out=w3:errorcluster)  [unwired: 1 in, 2 out]
  n119 = call "Teardown Framework.vi"("error in (no error)"=w3) -> ("error out"=→"error out":errorcluster)  [unwired: 10 in]
